vi "Scope Analysis V2.vi"() -> ()   [LabVIEW 2016]
panel:
  out "Point (Max)":dbl format="%#_13g"
  out "Contrast (Max)":dbl format="%#_13g"
  out "XY-Graph":cluster{dbl[], dbl[]}[](graph)
  out "Waveform Graph":dbl[][](graph)
  in  "Start Point":i32
  in  "Signal Length":i32
  in  "Instructions":string
  in  "Path of Folder":path
  in  "Index #":dbl(slide) step=1.0 scale=1.0..110.0
  # "Index # - Selects the .dat file with the index # chosen (ie. If 3 is selected on the slider, the .vi will graph 3_wav.dat)\n\nPath of Folder - User needs to select a file from the folder where the .dat file is located and then remove the title of .dat file so only the path\nof the folder remains (ie. C:\\Usr\\Name\\Folder_where_dat_files_are_located)"
  # "Signal Length is the length of the Integration Window"
  # "FUTURE UPDATES:\n\n-Length of index # scale adjusted so errors do not occur\n-Starting point for integration window \n-Average contrast analysis for the .dat files"
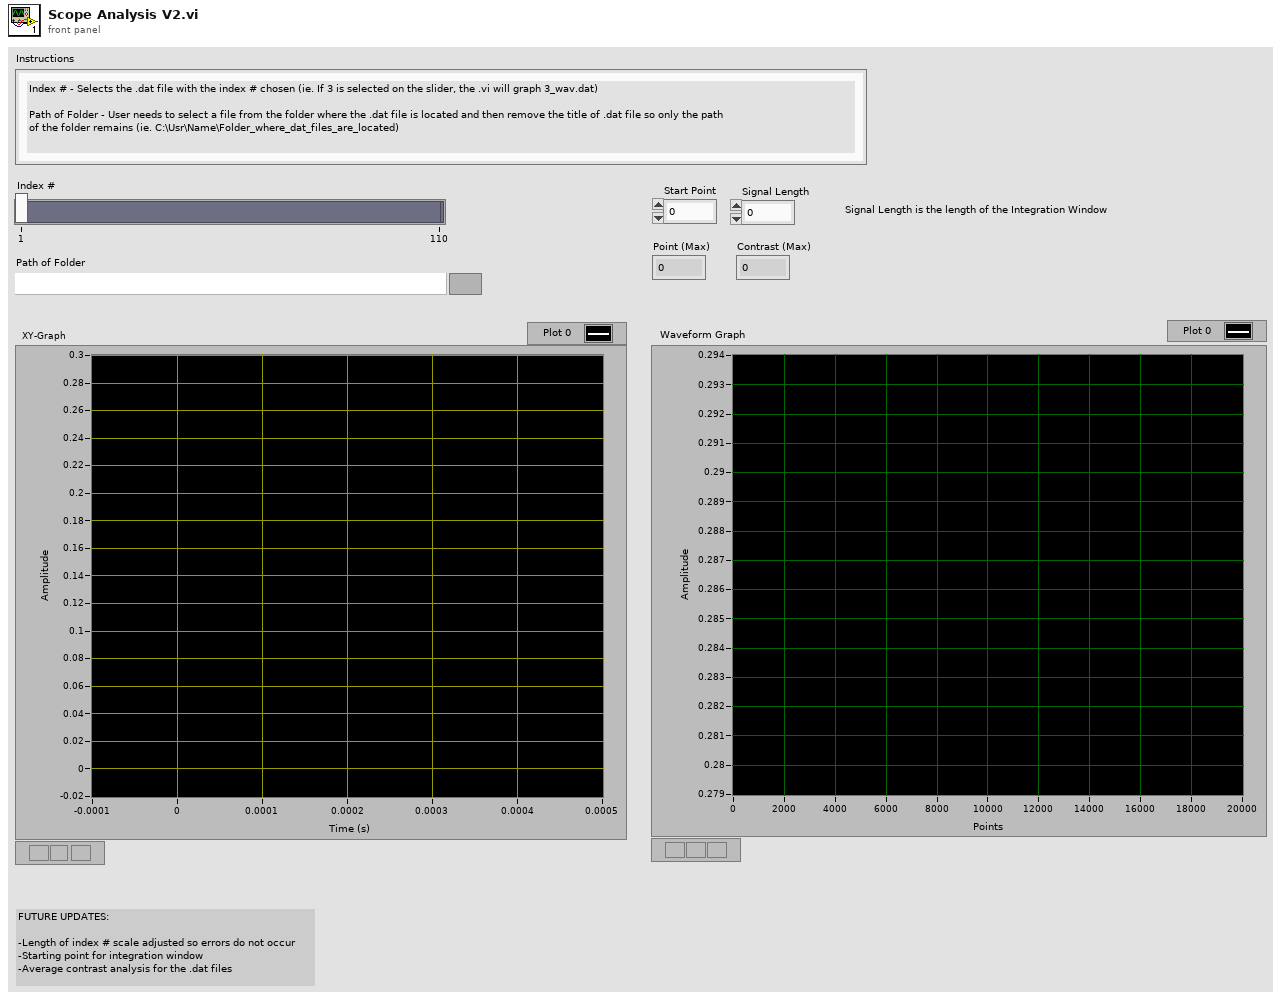
[diagram p1: front panel]
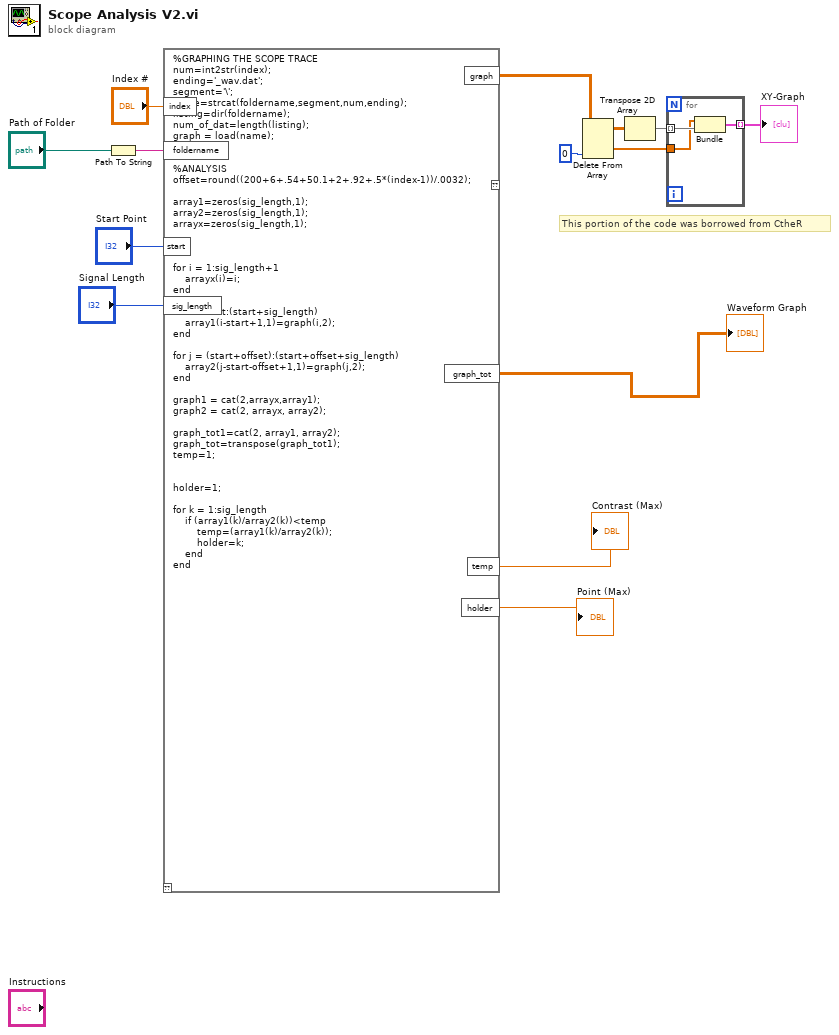
[diagram p0: block diagram]
diagram:
  # "This portion of the code was borrowed from CtheR"
  n1 = Path To String(path="Path of Folder") -> (string=w14:string)
  n2 = script code="%GRAPHING THE SCOPE TRACE\nnum=int2str(index);\nending='_wav.dat';\nsegment='\\';\nname=strcat(foldername,segment,num,ending);\nlisting=dir(foldername);\nnum_of_dat=length(listing);\ngraph = load(name);\n\n\n%ANALYSIS\noffset=round((200+6+.54+50.1+2+.92+.5*(index-1))/.0032);\n\narray1=zeros(sig_length,1);\narray2=zeros(sig_length,1);\narrayx=zeros(sig_length,1);\n\n\n\nfor i = 1:sig_length+1\n    arrayx(i)=i;\nend\n\nfor i =start:(start+sig_length)\n    array1(i-start+1,1)=graph(i,2);\nend\n\nfor j = (start+offset):(start+offset+sig_length)\n    array2(j-start-offset+1,1)=graph(j,2);\nend\n\ngraph1 = cat(2,arrayx,array1);\ngraph2 = cat(2, arrayx, array2);\n\ngraph_tot1=cat(2, array1, array2);\ngraph_tot=transpose(graph_tot1);\ntemp=1;\n\n\nholder=1;\n\nfor k = 1:sig_length\n    if (array1(k)/array2(k))<temp\n        temp=(array1(k)/array2(k));\n        holder=k;\n    end\nend"("index"="Index #", "foldername"=w14, "start"="Start Point", "sig_length"="Signal Length") -> ("graph"=w3:dbl[][], "graph_tot"=→"Waveform Graph":dbl[][], "temp"=→"Contrast (Max)":dbl, "holder"=→"Point (Max)":dbl)  [unwired: 1 in, 1 out]
  n3 = Delete From Array(array=w3, index (col)=0 ("Deaktivierter Index (Spalte)")) -> (deleted portion=w8:dbl[], array with subset deleted=w6:dbl[][])  [unwired: 2 in]
  n4 = Transpose 2D Array(2D array=w6) -> (transposed array=w5:dbl[][])
  n5 = for {
    tunnel: w8 -> [w16]
    tunnel: w5 -> [w17] mode=indexing
    tunnel: [w15] -> w7 mode=indexing
    n6 = Bundle(w16, w17) -> (w15:cluster{dbl[], dbl[]})  [unwired: 1 in]
  }
  "XY-Graph" <- w7
